vi "Load CHM.vi"(8 "error in (no error)":errorcluster, 10 "HTML File to Load":string, 11 "Main CHM File":string) -> (0 "error out":errorcluster)   [LabVIEW 2020, in "SEECD System Explorer.lvlib"]
uses:
  SEECD System Explorer.lvlib
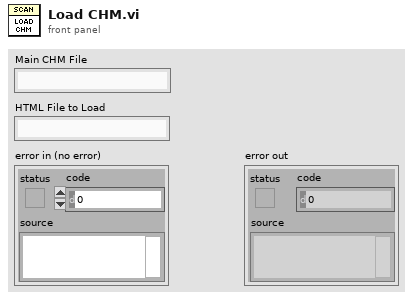
[diagram p1: front panel]
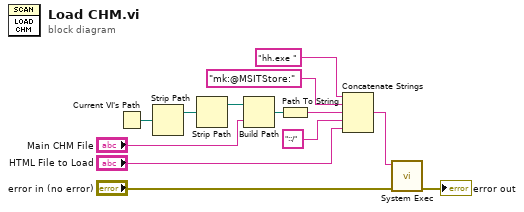
[diagram p0: block diagram]
diagram:
  n1 = Current VI's Path() -> (path=w12:path)
  n2 = Strip Path(path=w12) -> (stripped path=w11:path)  [unwired: 1 out]
  n3 = Strip Path(path=w11) -> (stripped path=w6:path)  [unwired: 1 out]
  n4 = Build Path(base path=w6, name or relative path="Main CHM File") -> (appended path=w8:path)
  n5 = Path To String(path=w8) -> (string=w9:string)
  n6 = Concatenate Strings("hh.exe " ("string"), "mk:@MSITStore:" ("string"), w9, "::/" ("name or relative path"), "HTML File to Load") -> (w1:string)
  n7 = call <vilib>:"System Exec.vi"("error in (no error)"="error in (no error)", "command line"=w1) -> ("error out"=→"error out":errorcluster)  [unwired: 6 in, 3 out]
